vi "Get Table Row by Index (VAR).vi"(7 "Sheet Name":string, 8 "error in":errorcluster, 9 "Row Index":i32, 10 "Table Name":string, 11 "SpreadsheetDoc in":refnum<k24>) -> (0 "error out":errorcluster, 2 "Rows":variant[](array[variant]), 3 "SpreadsheetDoc out":refnum<k24>)   [LabVIEW 2019, in "Open Xml.lvlib"]
uses:
  Open Xml.lvlib
  D:/git/Open-Xml-LabVIEW/Source/DocumentFormat.OpenXml.dll
  DocumentFormat.OpenXml.dll
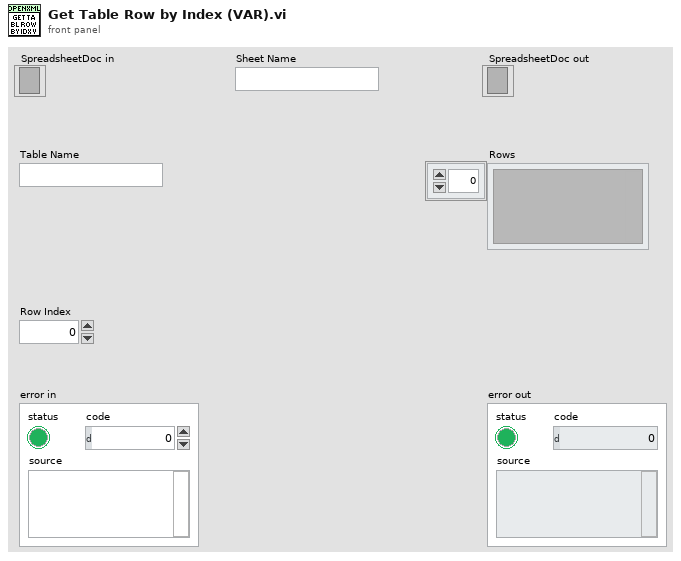
[diagram p1: front panel]
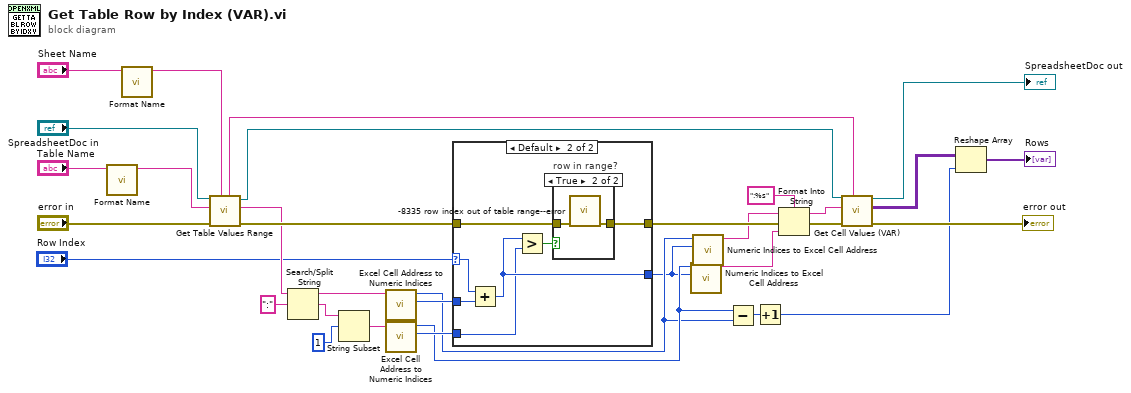
[diagram p0: block diagram]
diagram:
  n1 = call "Format Name.vi"("Sheet Name"="Table Name") -> ("Formatted Sheet Name"=w2:string)  [unwired: 10 in]
  n2 = call "Format Name.vi"("Sheet Name"="Sheet Name") -> ("Formatted Sheet Name"=w1:string)  [unwired: 10 in]
  n3 = call "Get Table Values Range.vi"("Sheet Name in"=w1, "error in"="error in", "Table Name"=w2, "SpreadsheetDoc in"="SpreadsheetDoc in") -> ("error out"=w28:errorcluster, "Range"=w23:string, "SpreadsheetDoc out"=w27:refnum<k24>, "Sheet Name out"=w25:string)  [unwired: 4 in]
  n4 = Search/Split String(string=w23, search string/char (-)=":") -> (substring before match=w21:string, match + rest of string=w20:string)  [unwired: 1 in, 1 out]
  n5 = String Subset(string=w20, offset (0)=1) -> (substring=w18:string)  [unwired: 1 in]
  n6 = call "Excel Cell Address to Numeric Indices.vi"("Cell Name"=w21) -> ("Row Number"=w17:i32, "Column Number"=w4:i32)  [unwired: 9 in]
  n7 = call "Excel Cell Address to Numeric Indices.vi"("Cell Name"=w18) -> ("Row Number"=w14:i32, "Column Number"=w5:i32)  [unwired: 9 in]
  n8 = case shown="Default" "Row Index" {
    selector: "Row Index" -> [_ w40]
    tunnel: w28 -> [w35 w42]
    tunnel: w17 -> [_ w41]
    tunnel: [w35 w39] -> w11
    tunnel: w14 -> [w34 w36]
    tunnel: [w34 w37] -> w3
    frame ..-1 {
    }
    frame Default {
      n9 = Add(x=w40, y=w41) -> (x+y=w37:i32)
      n10 = Greater?(x=w37, y=w36) -> (0:w38:bool)
      n11 = case "row in range?" shown="True" w38 {
        tunnel: w42 -> [w43 w45]
        tunnel: [w43 w44] -> w39
        frame False {
        }
        frame True {
          n12 = call "-8335 row index out of table range--error.vi"("error in"=w45) -> ("error out"=w44:errorcluster)  [unwired: 9 in, 1 out]
        }
      }
    }
  }
  n13 = call "Numeric Indices to Excel Cell Address.vi"("Row"=w3, "Column"=w5) -> ("Cell Address"=w9:string)  [unwired: 9 in]
  n14 = call "Numeric Indices to Excel Cell Address.vi"("Row"=w3, "Column"=w4) -> ("Cell Address"=w8:string)  [unwired: 9 in]
  n15 = Subtract(x=w5, y=w4) -> (x-y=w7:i32)
  n16 = Increment(x=w7) -> (x+1=w6:i32)
  n17 = Format Into String(format string=":%s", initial string=w8, error in=w11, w9) -> (resulting string=w12:string, error out=w10:errorcluster)
  n18 = call "Get Cell Values (VAR).vi"("Sheet Name in"=w25, "error in"=w10, "Cell Range"=w12, "SpreadsheetDoc in"=w27) -> ("error out"=→"error out":errorcluster, "Cell Values"=w31:variant[][], "SpreadsheetDoc out"=→"SpreadsheetDoc out":refnum<k24>)  [unwired: 5 in]
  n19 = Reshape Array(w31, w6) -> (→"Rows":variant[])
